vi "字母键盘.vi"() -> (1 "字符串":string, 2 "取消标志":bool)   [LabVIEW 2009]
panel:
  in  "esc":bool
  in  "下划线":bool
  in  "-":bool
  in  "逗号":bool
  out "数据是否有效":bool=TRUE
  out "是否大写":bool caption="大写"
  in  "大写":bool
  in  "后退":bool
  in  "清空":bool
  in  "取消":bool
  in  "确定":bool
  in  "0":bool
  in  "9":bool
  in  "8":bool
  in  "7":bool
  in  "6":bool
  in  "5":bool
  in  "4":bool
  in  "3":bool
  in  "2":bool
  in  "1":bool
  in  "N":bool
  in  "Z":bool
  in  "Y":bool
  in  "X":bool
  in  "W":bool
  in  "V":bool
  in  "U":bool
  in  "T":bool
  in  "S":bool
  in  "R":bool
  in  "Q":bool
  in  "P":bool
  in  "O":bool
  in  "M":bool
  in  "L":bool
  in  "K":bool
  in  "J":bool
  in  "I":bool
  in  "H":bool
  in  "G":bool
  in  "F":bool
  in  "E":bool
  in  "D":bool
  in  "C":bool
  in  "B":bool
  in  "A":bool
  # "输入数据:"
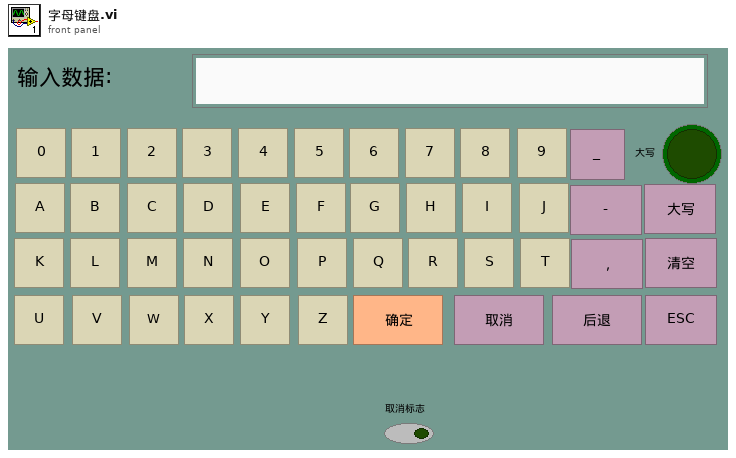
[diagram p1: front panel]
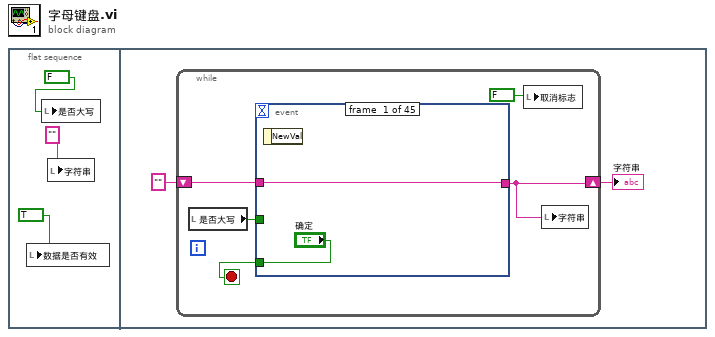
[diagram p0: block diagram]
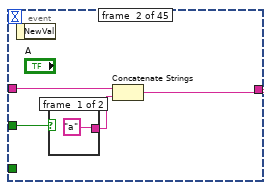
[diagram p2: hidden frame]
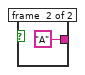
[diagram p3: hidden frame]
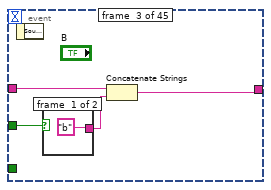
[diagram p4: hidden frame]
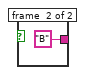
[diagram p5: hidden frame]
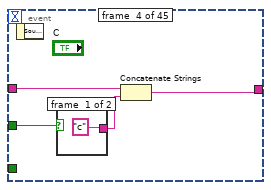
[diagram p6: hidden frame]
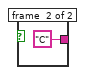
[diagram p7: hidden frame]
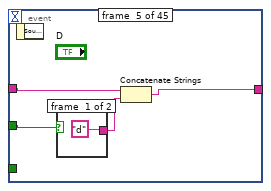
[diagram p8: hidden frame]
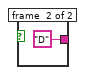
[diagram p9: hidden frame]
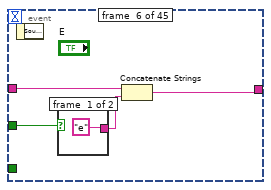
[diagram p10: hidden frame]
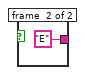
[diagram p11: hidden frame]
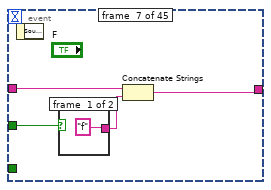
[diagram p12: hidden frame]
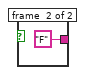
[diagram p13: hidden frame]
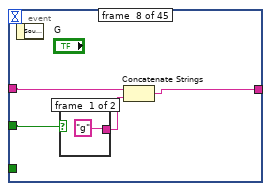
[diagram p14: hidden frame]
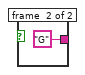
[diagram p15: hidden frame]
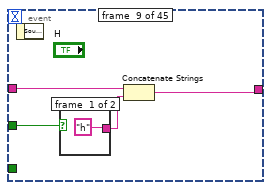
[diagram p16: hidden frame]
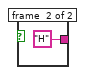
[diagram p17: hidden frame]
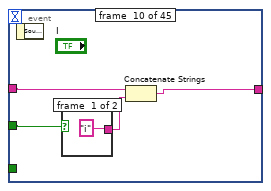
[diagram p18: hidden frame]
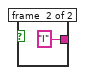
[diagram p19: hidden frame]
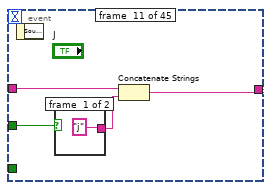
[diagram p20: hidden frame]
diagram:
  n1 = flat-sequence {
    frame #0 {
      n2 = local write "数据是否有效"(TRUE ("数据是否有效")) -> ()
      n3 = local write "是否大写"(FALSE ("大写")) -> ()
      n4 = local write "字符串"("" ("字符串")) -> ()
    }
    frame #1 {
      n5 = while {
        shift-right: [w7] -> w4
        shift-left: "" ("字符串") -> [w9]
        stop <- w8 stop-if-true
        n6 = local read "是否大写"() -> (w10:bool)
        n7 = event shown="[44] \"取消\": 值改变" {
          selector: _ -> [_ _ _ _ _ _ _ _ _ _ _ _ _ _ _ _ _ _ _ _ _ _ _ _ _ _ _ _ _ _ _ _ _ _ _ _ _ _ _ _ _ _ _ _ _]
          dyn-events: _ -> [_ _ _ _ _ _ _ _ _ _ _ _ _ _ _ _ _ _ _ _ _ _ _ _ _ _ _ _ _ _ _ _ _ _ _ _ _ _ _ _ _ _ _ _ _]
          timeout: _ -> [_ _ _ _ _ _ _ _ _ _ _ _ _ _ _ _ _ _ _ _ _ _ _ _ _ _ _ _ _ _ _ _ _ _ _ _ _ _ _ _ _ _ _ _ _]
          tunnel: w10 -> [_ w16 w20 w26 w32 w38 w44 w50 w56 w62 w68 w74 w80 w86 w92 w98 w104 w110 w116 w122 w128 w134 w140 w146 w152 w158 w164 _ _ _ _ _ _ _ _ _ _ _ _ _ _ _ _ _ _]
          tunnel: w9 -> [w11 w14 w21 w27 w33 w39 w45 w51 w57 w63 w69 w75 w81 w87 w93 w99 w105 w111 w117 w123 w129 w135 w141 w147 w153 w159 w165 w169 w173 w176 w179 w182 w185 w188 w191 w194 w197 w200 _ w206 w209 w211 _ w219 _]
          tunnel: ["确定" _ _ _ _ _ _ _ _ _ _ _ _ _ _ _ _ _ _ _ _ _ _ _ _ _ _ _ _ _ _ _ _ _ _ _ _ _ TRUE ("确定") _ _ _ _ _ TRUE ("确定")] -> w8
          tunnel: [w11 w13 w19 w25 w31 w37 w43 w49 w55 w61 w67 w73 w79 w85 w91 w97 w103 w109 w115 w121 w127 w133 w139 w145 w151 w157 w163 w170 w172 w175 w178 w181 w184 w187 w190 w193 w196 w199 _ w205 w208 w211 "" ("字符串") w216 _] -> w7
          event #0 {
            n8 = event-data() -> ()  [unwired: 1 in, 1 out]
          }
          event #1 {
            n9 = event-data() -> ()  [unwired: 1 in, 1 out]
            n10 = case shown="真" w16 {
              tunnel: ["a" ("字符串") "A" ("字符串")] -> w15
              frame #0 {
              }
              frame #1 {
              }
            }
            n11 = Concatenate Strings(w14, w15) -> (w13:string)
          }
          event #2 {
            n12 = event-data() -> ()  [unwired: 1 in, 1 out]
            n13 = case shown="真" w20 {
              tunnel: ["b" ("字符串") "B" ("字符串")] -> w22
              frame #0 {
              }
              frame #1 {
              }
            }
            n14 = Concatenate Strings(w21, w22) -> (w19:string)
          }
          event #3 {
            n15 = event-data() -> ()  [unwired: 1 in, 1 out]
            n16 = case shown="真" w26 {
              tunnel: ["c" ("字符串") "C" ("字符串")] -> w28
              frame #0 {
              }
              frame #1 {
              }
            }
            n17 = Concatenate Strings(w27, w28) -> (w25:string)
          }
          event #4 {
            n18 = event-data() -> ()  [unwired: 1 in, 1 out]
            n19 = case shown="真" w32 {
              tunnel: ["d" ("字符串") "D" ("字符串")] -> w34
              frame #0 {
              }
              frame #1 {
              }
            }
            n20 = Concatenate Strings(w33, w34) -> (w31:string)
          }
          event #5 {
            n21 = event-data() -> ()  [unwired: 1 in, 1 out]
            n22 = case shown="真" w38 {
              tunnel: ["e" ("字符串") "E" ("字符串")] -> w40
              frame #0 {
              }
              frame #1 {
              }
            }
            n23 = Concatenate Strings(w39, w40) -> (w37:string)
          }
          event #6 {
            n24 = event-data() -> ()  [unwired: 1 in, 1 out]
            n25 = case shown="真" w44 {
              tunnel: ["f" ("字符串") "F" ("字符串")] -> w46
              frame #0 {
              }
              frame #1 {
              }
            }
            n26 = Concatenate Strings(w45, w46) -> (w43:string)
          }
          event #7 {
            n27 = event-data() -> ()  [unwired: 1 in, 1 out]
            n28 = case shown="假" w50 {
              tunnel: ["g" ("字符串") "G" ("字符串")] -> w52
              frame #0 {
              }
              frame #1 {
              }
            }
            n29 = Concatenate Strings(w51, w52) -> (w49:string)
          }
          event #8 {
            n30 = event-data() -> ()  [unwired: 1 in, 1 out]
            n31 = case shown="假" w56 {
              tunnel: ["h" ("字符串") "H" ("字符串")] -> w58
              frame #0 {
              }
              frame #1 {
              }
            }
            n32 = Concatenate Strings(w57, w58) -> (w55:string)
          }
          event #9 {
            n33 = event-data() -> ()  [unwired: 1 in, 1 out]
            n34 = case shown="真" w62 {
              tunnel: ["i" ("字符串") "I" ("字符串")] -> w64
              frame #0 {
              }
              frame #1 {
              }
            }
            n35 = Concatenate Strings(w63, w64) -> (w61:string)
          }
          event #10 {
            n36 = event-data() -> ()  [unwired: 1 in, 1 out]
            n37 = case shown="真" w68 {
              tunnel: ["j" ("字符串") "J" ("字符串")] -> w70
              frame #0 {
              }
              frame #1 {
              }
            }
            n38 = Concatenate Strings(w69, w70) -> (w67:string)
          }
          event #11 {
            n39 = event-data() -> ()  [unwired: 1 in, 1 out]
            n40 = case shown="真" w74 {
              tunnel: ["k" ("字符串") "K" ("字符串")] -> w76
              frame #0 {
              }
              frame #1 {
              }
            }
            n41 = Concatenate Strings(w75, w76) -> (w73:string)
          }
          event #12 {
            n42 = event-data() -> ()  [unwired: 1 in, 1 out]
            n43 = case shown="真" w80 {
              tunnel: ["l" ("字符串") "L" ("字符串")] -> w82
              frame #0 {
              }
              frame #1 {
              }
            }
            n44 = Concatenate Strings(w81, w82) -> (w79:string)
          }
          event #13 {
            n45 = event-data() -> ()  [unwired: 1 in, 1 out]
            n46 = case shown="真" w86 {
              tunnel: ["m" ("字符串") "M" ("字符串")] -> w88
              frame #0 {
              }
              frame #1 {
              }
            }
            n47 = Concatenate Strings(w87, w88) -> (w85:string)
          }
          event #14 {
            n48 = event-data() -> ()  [unwired: 1 in, 1 out]
            n49 = case shown="真" w92 {
              tunnel: ["n" ("字符串") "N" ("字符串")] -> w94
              frame #0 {
              }
              frame #1 {
              }
            }
            n50 = Concatenate Strings(w93, w94) -> (w91:string)
          }
          event #15 {
            n51 = event-data() -> ()  [unwired: 1 in, 1 out]
            n52 = case shown="真" w98 {
              tunnel: ["o" ("字符串") "O" ("字符串")] -> w100
              frame #0 {
              }
              frame #1 {
              }
            }
            n53 = Concatenate Strings(w99, w100) -> (w97:string)
          }
          event #16 {
            n54 = event-data() -> ()  [unwired: 1 in, 1 out]
            n55 = case shown="真" w104 {
              tunnel: ["p" ("字符串") "P" ("字符串")] -> w106
              frame #0 {
              }
              frame #1 {
              }
            }
            n56 = Concatenate Strings(w105, w106) -> (w103:string)
          }
          event #17 {
            n57 = event-data() -> ()  [unwired: 1 in, 1 out]
            n58 = case shown="真" w110 {
              tunnel: ["q" ("字符串") "Q" ("字符串")] -> w112
              frame #0 {
              }
              frame #1 {
              }
            }
            n59 = Concatenate Strings(w111, w112) -> (w109:string)
          }
          event #18 {
            n60 = event-data() -> ()  [unwired: 1 in, 1 out]
            n61 = case shown="真" w116 {
              tunnel: ["r" ("字符串") "R" ("字符串")] -> w118
              frame #0 {
              }
              frame #1 {
              }
            }
            n62 = Concatenate Strings(w117, w118) -> (w115:string)
          }
          event #19 {
            n63 = event-data() -> ()  [unwired: 1 in, 1 out]
            n64 = case shown="真" w122 {
              tunnel: ["s" ("字符串") "S" ("字符串")] -> w124
              frame #0 {
              }
              frame #1 {
              }
            }
            n65 = Concatenate Strings(w123, w124) -> (w121:string)
          }
          event #20 {
            n66 = event-data() -> ()  [unwired: 1 in, 1 out]
            n67 = case shown="假" w128 {
              tunnel: ["t" ("字符串") "T" ("字符串")] -> w130
              frame #0 {
              }
              frame #1 {
              }
            }
            n68 = Concatenate Strings(w129, w130) -> (w127:string)
          }
          event #21 {
            n69 = event-data() -> ()  [unwired: 1 in, 1 out]
            n70 = case shown="真" w134 {
              tunnel: ["u" ("字符串") "U" ("字符串")] -> w136
              frame #0 {
              }
              frame #1 {
              }
            }
            n71 = Concatenate Strings(w135, w136) -> (w133:string)
          }
          event #22 {
            n72 = event-data() -> ()  [unwired: 1 in, 1 out]
            n73 = case shown="真" w140 {
              tunnel: ["v" ("字符串") "V" ("字符串")] -> w142
              frame #0 {
              }
              frame #1 {
              }
            }
            n74 = Concatenate Strings(w141, w142) -> (w139:string)
          }
          event #23 {
            n75 = event-data() -> ()  [unwired: 1 in, 1 out]
            n76 = case shown="真" w146 {
              tunnel: ["w" ("字符串") "W" ("字符串")] -> w148
              frame #0 {
              }
              frame #1 {
              }
            }
            n77 = Concatenate Strings(w147, w148) -> (w145:string)
          }
          event #24 {
            n78 = event-data() -> ()  [unwired: 1 in, 1 out]
            n79 = case shown="假" w152 {
              tunnel: ["x" ("字符串") "X" ("字符串")] -> w154
              frame #0 {
              }
              frame #1 {
              }
            }
            n80 = Concatenate Strings(w153, w154) -> (w151:string)
          }
          event #25 {
            n81 = event-data() -> ()  [unwired: 1 in, 1 out]
            n82 = case shown="假" w158 {
              tunnel: ["y" ("字符串") "Y" ("字符串")] -> w160
              frame #0 {
              }
              frame #1 {
              }
            }
            n83 = Concatenate Strings(w159, w160) -> (w157:string)
          }
          event #26 {
            n84 = event-data() -> ()  [unwired: 1 in, 1 out]
            n85 = case shown="真" w164 {
              tunnel: ["z" ("字符串") "Z" ("字符串")] -> w166
              frame #0 {
              }
              frame #1 {
              }
            }
            n86 = Concatenate Strings(w165, w166) -> (w163:string)
          }
          event #27 {
            n87 = event-data() -> ()  [unwired: 1 in, 1 out]
            n88 = Concatenate Strings(w169, "0" ("字符串")) -> (w170:string)
          }
          event #28 {
            n89 = event-data() -> ()  [unwired: 1 in, 1 out]
            n90 = Concatenate Strings(w173, "1" ("字符串")) -> (w172:string)
          }
          event #29 {
            n91 = event-data() -> ()  [unwired: 1 in, 1 out]
            n92 = Concatenate Strings(w176, "2" ("字符串")) -> (w175:string)
          }
          event #30 {
            n93 = event-data() -> ()  [unwired: 1 in, 1 out]
            n94 = Concatenate Strings(w179, "3" ("字符串")) -> (w178:string)
          }
          event #31 {
            n95 = event-data() -> ()  [unwired: 1 in, 1 out]
            n96 = Concatenate Strings(w182, "4" ("字符串")) -> (w181:string)
          }
          event #32 {
            n97 = event-data() -> ()  [unwired: 1 in, 1 out]
            n98 = Concatenate Strings(w185, "5" ("字符串")) -> (w184:string)
          }
          event #33 {
            n99 = event-data() -> ()  [unwired: 1 in, 1 out]
            n100 = Concatenate Strings(w188, "6" ("字符串")) -> (w187:string)
          }
          event #34 {
            n101 = event-data() -> ()  [unwired: 1 in, 1 out]
            n102 = Concatenate Strings(w191, "7" ("字符串")) -> (w190:string)
          }
          event #35 {
            n103 = event-data() -> ()  [unwired: 1 in, 1 out]
            n104 = Concatenate Strings(w194, "8" ("字符串")) -> (w193:string)
          }
          event #36 {
            n105 = event-data() -> ()  [unwired: 1 in, 1 out]
            n106 = Concatenate Strings(w197, "9" ("字符串")) -> (w196:string)
          }
          event #37 {
            n107 = event-data() -> ()  [unwired: 1 in, 1 out]
            n108 = Concatenate Strings(w200, "," ("字符串")) -> (w199:string)
          }
          event #38 {
            n109 = event-data() -> ()  [unwired: 1 in, 1 out]
            n110 = local write "数据是否有效"(FALSE ("数据是否有效")) -> ()
            n111 = local write "取消标志"(TRUE ("取消标志")) -> ()
          }
          event #39 {
            n112 = event-data() -> ()  [unwired: 1 in, 1 out]
            n113 = Concatenate Strings(w206, "-" ("字符串")) -> (w205:string)
          }
          event #40 {
            n114 = event-data() -> ()  [unwired: 1 in, 1 out]
            n115 = Concatenate Strings(w209, "_" ("字符串")) -> (w208:string)
          }
          event #41 {
            n116 = event-data() -> ()  [unwired: 1 in, 1 out]
            n117 = local read "是否大写"() -> (w212:bool)
            n118 = case shown="真" w212 {
              frame #0 {
                n119 = local write "是否大写"(TRUE ("是否大写")) -> ()
              }
              frame #1 {
                n120 = local write "是否大写"(FALSE ("是否大写")) -> ()
              }
            }
          }
          event #42 {
            n121 = event-data() -> ()  [unwired: 1 in, 1 out]
          }
          event #43 {
            n122 = event-data() -> ()  [unwired: 1 in, 1 out]
            n123 = String Length(string=w219) -> (length=w217:i32)
            n124 = Decrement(x=w217) -> (x-1=w218:i32)
            n125 = String Subset(string=w219, length (rest)=w218) -> (substring=w216:string)  [unwired: 1 in]
          }
          event #44 {
            n126 = event-data() -> ()  [unwired: 1 in, 1 out]
            "数据是否有效" <- FALSE ("数据是否有效")
            "取消标志" <- TRUE ("取消标志")
          }
        }
        n127 = local write "取消标志"(FALSE ("取消标志")) -> ()
        n128 = local write "字符串"(w7) -> ()
      }
      "字符串" <- w4
    }
  }
